vi "Init Motor Config Obj.vi"(8 "error in (no error)":errorcluster, 11 "VacuumLine Configuration in":refnum<class "VacuumLine Configuration.lvclass">) -> (0 "error out":errorcluster, 2 "Motor Config Obj":refnum<class "Motor Configuration.lvclass">, 3 "VacuumLine Configuration out":refnum<class "VacuumLine Configuration.lvclass">)   [LabVIEW 2016, in "Hardware.lvlib" / "VacuumLine.lvlib" / "VacuumLine Configuration.lvclass"]
uses:
  <userlib>/Common Components/Hardware/Abstract System/VacuumLine/VacuumLine Config/VacuumLine Configuration.lvclass
  C:/Program Files (x86)/National Instruments/LabVIEW 2016/user.lib/Configuration Dialog Actor/Configuration.lvclass
  <userlib>/Common Components/Hardware/Motor/Motor Config/Motor Configuration.lvclass
  <userlib>/Common Components/Hardware/Motor/Motor Config/Motor Configuration.lvclass/Motor Configuration.ctl
  <userlib>/Common Components/Hardware/Abstract System/VacuumLine/VacuumLine Config/VacuumLine Configuration.lvclass/VacuumLine Configuration.ctl
  <userlib>/Configuration Dialog Actor/Configuration.lvclass/Configuration.ctl
  <userlib>/Common Components/Hardware/Abstract System/VacuumLine/VacuumLine/VacuumLine.lvclass/VacuumLine.ctl
  <userlib>/Common Components/Hardware/Abstract System/VacuumLine/VacuumLine Config/Accessors/Read VacuumLine Obj.vi
  <userlib>/Configuration Dialog Actor/Accessors/Read Change Display.vi
  <userlib>/Configuration Dialog Actor/Accessors/Read Sub Panel.vi
  <userlib>/Configuration Dialog Actor/Accessors/Read Title.vi
  <userlib>/Configuration Dialog Actor/Accessors/Read Categories.vi
  <userlib>/Configuration Dialog Actor/Accessors/Write Change Display.vi
  <userlib>/Configuration Dialog Actor/Accessors/Write Sub Panel.vi
  <userlib>/Configuration Dialog Actor/Accessors/Write Title.vi
  <userlib>/Configuration Dialog Actor/Accessors/Write Categories.vi
  <userlib>/Common Components/Hardware/Abstract System/VacuumLine/VacuumLine/VacuumLine.lvclass
  <userlib>/Common Components/Hardware/Motor/Motor/Motor.lvclass
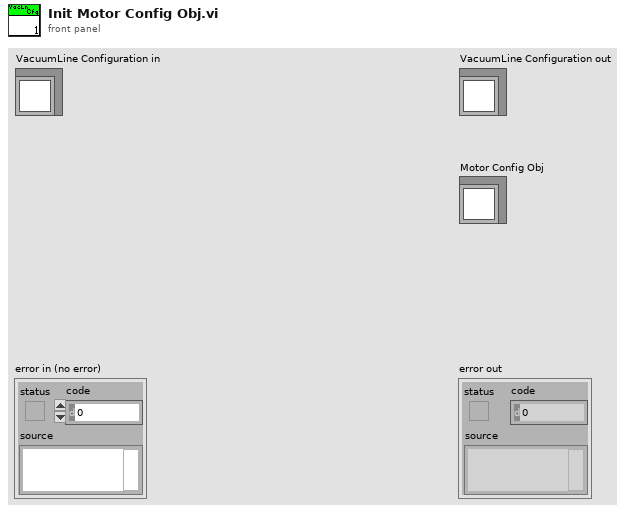
[diagram p1: front panel]
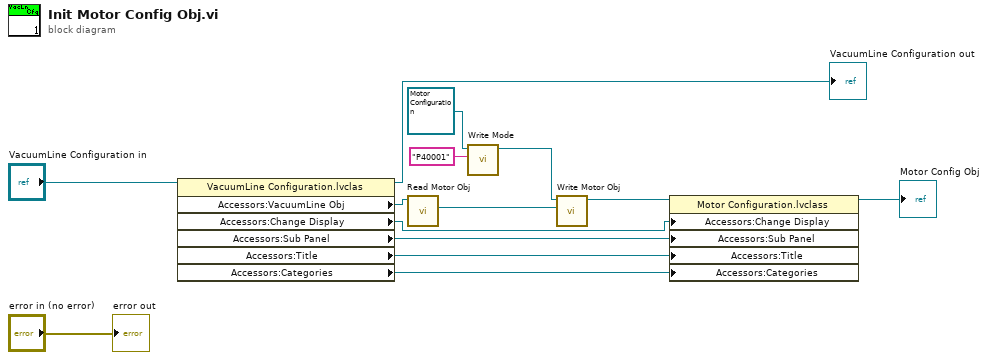
[diagram p0: block diagram]
diagram:
  n1 = property class="VacuumLine Configuration.lvclas"(reference="VacuumLine Configuration in") -> (reference out=→"VacuumLine Configuration out":refnum<class "VacuumLine Configuration.lvclass">, "Accessors:VacuumLine Obj"=w9:refnum<class "VacuumLine.lvclass">, "Accessors:Change Display"=w13:refnum<user-event>, "Accessors:Sub Panel"=w12:refnum<vi>, "Accessors:Title"=w11:refnum<vi>, "Accessors:Categories"=w10:refnum<vi>)  [unwired: 1 in, 1 out]
  n2 = call <userlib>:"Read Motor Obj.vi"("VacuumLine in"=w9) -> ("Hardware.lvlib:Motor.lvlib:Motor.lvclass"=w6:refnum<class "Motor.lvclass">)  [unwired: 8 in, 2 out]
  n3 = call <userlib>:"Write Mode.vi"("Mode"="P40001", "Motor Configuration in"=refnum<class "Motor Configuration.lvclass"> refnum ("Motor Config Obj")) -> ("Motor Configuration out"=w2:refnum<class "Motor Configuration.lvclass">)  [unwired: 9 in]
  n4 = call <userlib>:"Write Motor Obj.vi"("Hardware.lvlib:Motor.lvlib:Motor.lvclass"=w6, "Motor Configuration in"=w2) -> ("Motor Configuration out"=w5:refnum<class "Motor Configuration.lvclass">)  [unwired: 8 in, 1 out]
  n5 = property class="Motor Configuration.lvclass"(reference=w5, "Accessors:Change Display"=w13, "Accessors:Sub Panel"=w12, "Accessors:Title"=w11, "Accessors:Categories"=w10) -> (reference out=→"Motor Config Obj":refnum<class "Motor Configuration.lvclass">)  [unwired: 1 in, 1 out]
  "error out" <- "error in (no error)"
